vi "LaserError.vi"(9 "args":string[](array[string]), 10 "laserErrorType":T1) -> (0 "error out":errorcluster)   [LabVIEW 2016, in "Laser Diode Controller.lvlib" / "KLD101.lvclass"]
uses:
  KLD101.lvclass
  TypeDefs/KLD-LaserErrors.ctl
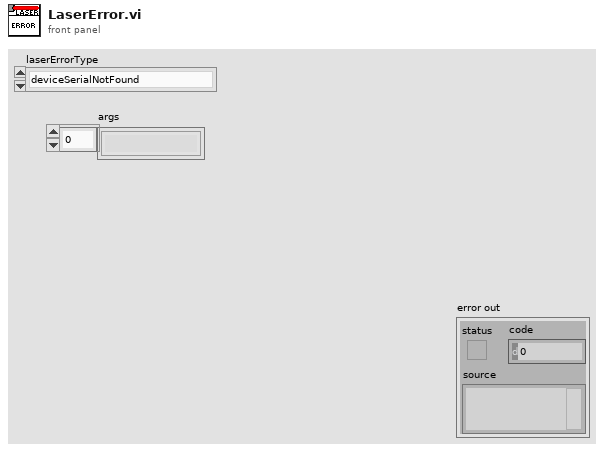
[diagram p1: front panel]
types:
  T1 = typedef "Laser Diode Controller.lvlib/KLD101.lvclass/KLD-LaserErrors.ctl" = enum16{"deviceSerialNotFound"}
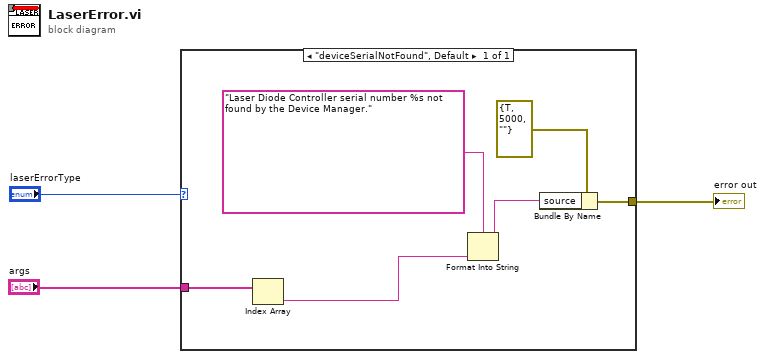
[diagram p0: block diagram]
diagram:
  n1 = case shown="\"deviceSerialNotFound\", Default" "laserErrorType" {
    tunnel: [w8] -> w2
    tunnel: "args" -> [w5]
    frame "deviceSerialNotFound", Default {
      n2 = Index Array(array=w5) -> (element=w4:string)  [unwired: 1 in]
      n3 = Format Into String(format string="Laser Diode Controller serial number %s not found by the Device Manager." ("source"), w4) -> (resulting string=w6:string)  [unwired: 2 in, 1 out]
      n4 = Bundle By Name(cluster=errorcluster {"status"=TRUE, "code"=5000, "source"=""} ("error out"), "source"=w6) -> (w8:errorcluster)
    }
  }
  "error out" <- w2
